vi "LEDC SWIR Main_2015LED.vi"(0 "LEDAD Port":refnum<visa-resource-name>="COM7", 1 "Light Meter Port":refnum<visa-resource-name>="COM4", 3 "Intensity Desired":dbl(slide) scale=0.0..100.0, 4 "Enable LED":u8(slide) scale=0.0..31.0, 5 "error in (no error)":errorcluster, 6 "Mode":T1, 7 "2015 LED":bool, 8 "Channel":enum16{"Chn1", "Chn2"}(ring), 9 "DPLM":bool, 10 "Unit":u16(ring) items=["nW/cm^2", "pW/cm^2"], 11 "Calibration File":path) -> (12 "In Progress":bool, 13 "Done":bool, 14 "LEDAD Port out":refnum<visa-resource-name>, 15 "Light Meter Port out":refnum<visa-resource-name>, 17 "Illum":dbl format="%#_4g", 18 "Variance":dbl format="%#_4g", 19 "error out":errorcluster)   [LabVIEW 2010]
uses:
  Projects/2015 Multiport/Type Definitions/CamMode_TypeDef.ctl
  <vilib>/Utility/file.llb/Read From Spreadsheet File (DBL).vi
panel:
  # "%"
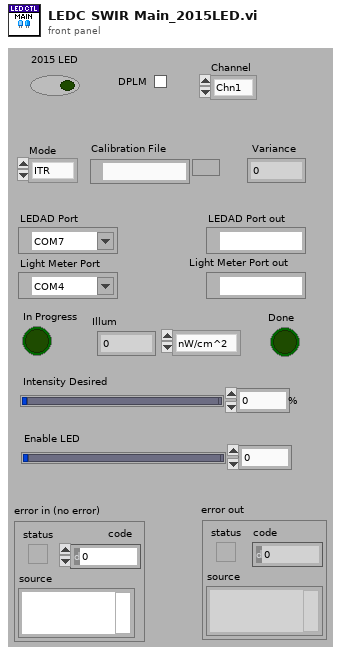
[diagram p1: front panel]
types:
  T1 = typedef "CamMode_TypeDef.ctl" = enum8{"ITR", "CDS", "IWR", "sCMOS"}
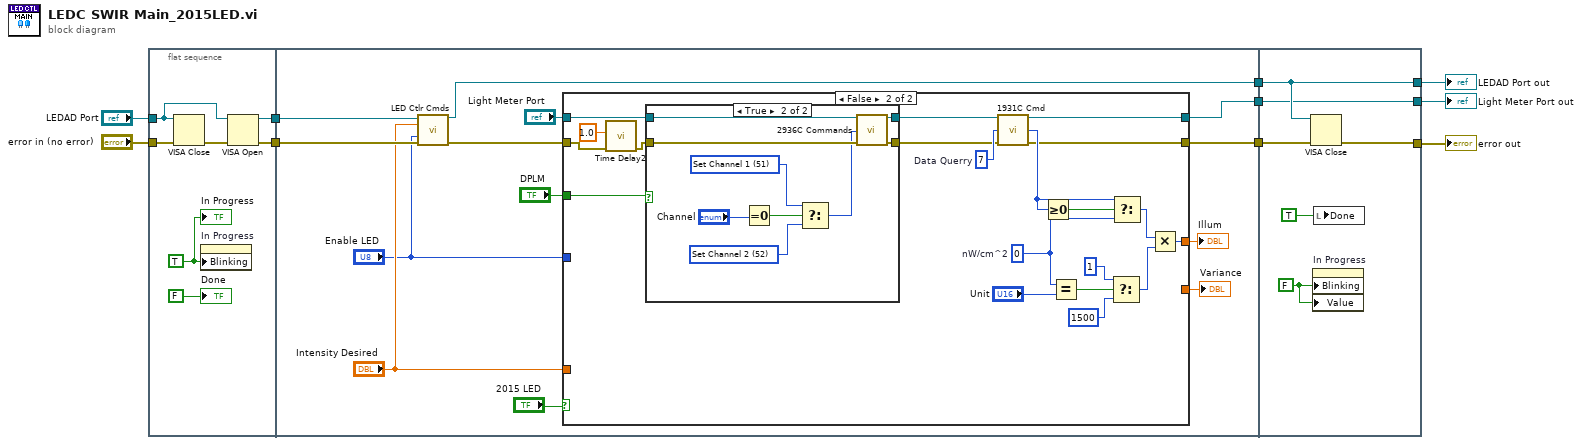
[diagram p0: block diagram]
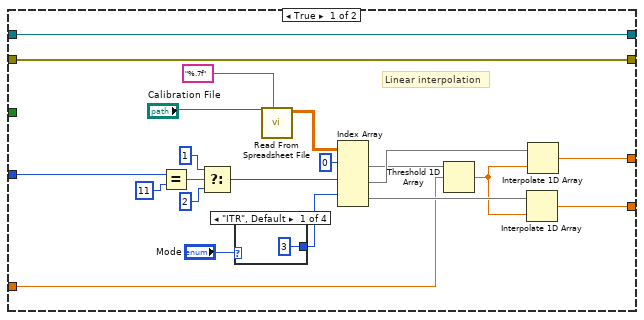
[diagram p2: hidden frame]
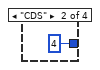
[diagram p3: hidden frame]
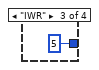
[diagram p4: hidden frame]
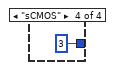
[diagram p5: hidden frame]
diagram:
  n1 = flat-sequence {
    tunnel: "LEDAD Port" -> [w13]
    tunnel: "error in (no error)" -> [w15]
    tunnel: [w14] -> w8
    tunnel: [w11] -> w1
    tunnel: w8 -> [w25]
    tunnel: [w27] -> w7
    tunnel: [w29] -> w6
    tunnel: [w23] -> w2
    tunnel: w1 -> [w24]
    tunnel: w7 -> [w91]
    tunnel: w6 -> [w89]
    tunnel: [w90] -> w3
    tunnel: [w89] -> w4
    tunnel: [w88] -> w5
    tunnel: w2 -> [w90]
    frame #0 {
      w12 = TRUE
      n2 = VISA Close(VISA resource name=w13, error in (no error)=w15) -> (error out=w16:errorcluster)
      n3 = property on="In Progress" class="Bool (strict)"("Blinking"=w12) -> ()  [unwired: 2 in, 2 out]
      n4 = VISA Open(error in (no error)=w16, VISA resource name=w13) -> (VISA resource name=w11:refnum<visa-resource-name>, error out=w14:errorcluster)  [unwired: 3 in]
      "Done" <- FALSE
      "In Progress" <- w12
    }
    frame #1 {
      n5 = call "LED Ctlr Cmds.vi"("VISA session"=w24, "Intensity"="Intensity Desired", "Enable"="Enable LED", "error in (no error)"=w25) -> ("VISA session out"=w23:refnum<visa-resource-name>, "error out"=w18:errorcluster)  [unwired: 7 in, 3 out]
      n6 = case shown="False" "2015 LED" {
        tunnel: w18 -> [w51 w57]
        tunnel: [w51 w65] -> w27
        tunnel: "Intensity Desired" -> [w36 _]
        tunnel: [w50 w63] -> w29
        tunnel: [w31 w64] -> w28
        tunnel: [w32 _] -> w26
        tunnel: "Light Meter Port" -> [w50 w60]
        tunnel: "DPLM" -> [_ w59]
        tunnel: "Enable LED" -> [w33 _]
        frame True {
          # "Linear interpolation"
          n7 = Equal?(x=w33, y=u8 11) -> (x = y?=w44:bool)
          n8 = Select(t=1 ("index (row)"), s=w44, f=2) -> (s? t:f=w45:i32)
          n9 = case shown="\"ITR\", Default" "Mode" {
            tunnel: [3 ("index") 4 ("index") 5 ("index") 3 ("index")] -> w48
            frame "ITR", Default {
            }
            frame "CDS" {
            }
            frame "IWR" {
            }
            frame "sCMOS" {
            }
          }
          n10 = call-poly <vilib>:"Read From Spreadsheet File.vi"("format (%.3f)"="%.7f", "file path (dialog if empty)"="Calibration File") -> ("all rows"=w39:dbl[][])  [unwired: 5 in, 4 out]
          n11 = Index Array(array=w39, index (row) #1=0 ("index (row)"), index (row) #2=w45, index (row) #3=w48) -> (element #1=w41:dbl[], element #2=w42:dbl[], element #3=w49:dbl[])  [unwired: 3 in]
          n12 = Threshold 1D Array(2:w36, 3:w41) -> (0:w43:dbl)  [unwired: 1 in]
          n13 = Interpolate 1D Array(1:w43, 2:w49) -> (0:w32:dbl)
          n14 = Interpolate 1D Array(1:w43, 2:w42) -> (0:w31:dbl)
        }
        frame False {
          w67 = 0  # nW/cm^2
          w71 = 7  # Data Querry
          n15 = call "Time Delay2"("error in (no error)"=w57, "Delay Time (s)"=1.0) -> ("error out"=w56:errorcluster)  [unwired: 9 in]
          n16 = case shown="True" w59 {
            tunnel: [w77 w86] -> w62
            tunnel: [w76 w85] -> w61
            tunnel: w56 -> [w77 w84]
            tunnel: w60 -> [w76 w83]
            frame False {
            }
            frame True {
              w80 = u16 52 items=["Attenuator OFF", "Attenuator ON", "Attenuator Query", "Beep OFF", "Beep ON", "Beep Query", "Clear Status Reg", "Get Power (nW)", "Echo OFF", "Echo ON", "Echo Query", "No Filter", "Analog Filter", "Digital FIlter", "Filter Query", "Hold", "Go", "Go Query", "Backlight OFF", "Backlight Medium", "Backlight High", "Backlight Query", "Set Dsplay Screen 0", "Set Display Screen 1", "Display Screen Query", "Mode DC Continuous", "Mode DC Single", "Mode Integrate", "Identification", "Auto Range", "Auto Range Query", "Signal Range 0", "Signal Range 1", "Signal Range 2", "Signal Range 3", "Signal Range 4", "Signal Range 5", "Signal Range 6", "Signal Range Query", "Store Reference", "Units W", "Units W/cm2", "Units dBm", "Units Joules", "Units Query", "Set Wavelength", "Wavelength Querry", "Mode Pesk-to-Peak Cont.", "Mode Peak-to-Peak Sing.", "Mode Query", "Channel Querry", "Set Channel 1", "Set Channel 2"] ("Command")
              w81 = u16 51 items=["Attenuator OFF", "Attenuator ON", "Attenuator Query", "Beep OFF", "Beep ON", "Beep Query", "Clear Status Reg", "Get Power (nW)", "Echo OFF", "Echo ON", "Echo Query", "No Filter", "Analog Filter", "Digital FIlter", "Filter Query", "Hold", "Go", "Go Query", "Backlight OFF", "Backlight Medium", "Backlight High", "Backlight Query", "Set Dsplay Screen 0", "Set Display Screen 1", "Display Screen Query", "Mode DC Continuous", "Mode DC Single", "Mode Integrate", "Identification", "Auto Range", "Auto Range Query", "Signal Range 0", "Signal Range 1", "Signal Range 2", "Signal Range 3", "Signal Range 4", "Signal Range 5", "Signal Range 6", "Signal Range Query", "Store Reference", "Units W", "Units W/cm2", "Units dBm", "Units Joules", "Units Query", "Set Wavelength", "Wavelength Querry", "Mode Pesk-to-Peak Cont.", "Mode Peak-to-Peak Sing.", "Mode Query", "Channel Querry", "Set Channel 1", "Set Channel 2"] ("Command")
              n17 = Equal To 0?(x="Channel") -> (x = 0?=w79:bool)
              n18 = Select(t=w81, s=w79, f=w80) -> (s? t:f=w78:u16)
              n19 = call "2936C Commands.vi"("Instrument Resource Name"=w83, "Command"=w78, "error in (no error)"=w84) -> ("VISA resource name out"=w85:refnum<visa-resource-name>, "error out"=w86:errorcluster)  [unwired: 8 in, 3 out]
            }
          }
          n20 = call "1931C Cmd.vi"("Instrument Resource Name"=w61, "Command"=w71, "error in (no error)"=w62) -> ("VISA resource name out"=w63:refnum<visa-resource-name>, "LM Response"=w68:i32, "error out"=w65:errorcluster)  [unwired: 8 in, 2 out]
          n21 = Greater Or Equal To 0?(x=w68) -> (x >= 0?=w69:bool)
          n22 = Equal?(x=w67, y="Unit") -> (x = y?=w73:bool)
          n23 = Select(t=1, s=w73, f=1500) -> (s? t:f=w72:i32)
          n24 = Select(t=w68, s=w69, f=w67) -> (s? t:f=w66:i32)
          n25 = Multiply(x=w66, y=w72) -> (x*y=w64:i32)
        }
      }
      "Illum" <- w28
      "Variance" <- w26
    }
    frame #2 {
      w87 = FALSE
      n26 = VISA Close(VISA resource name=w90, error in (no error)=w91) -> (error out=w88:errorcluster)
      n27 = property on="In Progress" class="Bool (strict)"("Blinking"=w87, "Value"=w87) -> ()  [unwired: 2 in, 2 out]
      n28 = local write "Done"(TRUE) -> ()
    }
  }
  "LEDAD Port out" <- w3
  "Light Meter Port out" <- w4
  "error out" <- w5
